vi "Control_motor.vi"() -> ()   [LabVIEW 2025]
uses:
  <vilib>/Instr/_visa.llb/VISA Configure Serial Port (Instr).vi
  <vilib>/addons/control/pid/pid.llb/PID (DBL).vi
  <vilib>/addons/control/pid/NI_PID_pid.lvlib
panel:
  out "Grados":dbl
  out "U":dbl format="%.2f"
  in  "Mandar Arduino":bool
  in  "Setpoint \nPosicion en grados":dbl
  in  "Kp":dbl=1.01
  in  "Ki":dbl=0.4
  in  "Kd":dbl=0.2
  in  "VISA resource name":refnum<visa-resource-name>
  out "Pulsos por vuelta":dbl
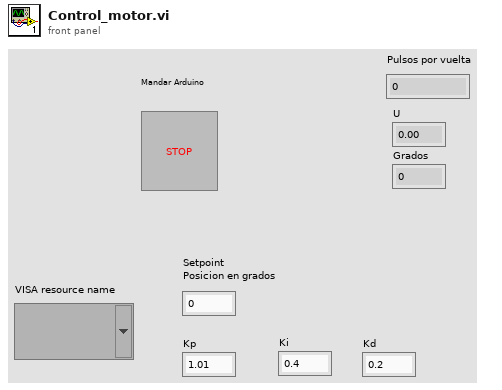
[diagram p1: front panel]
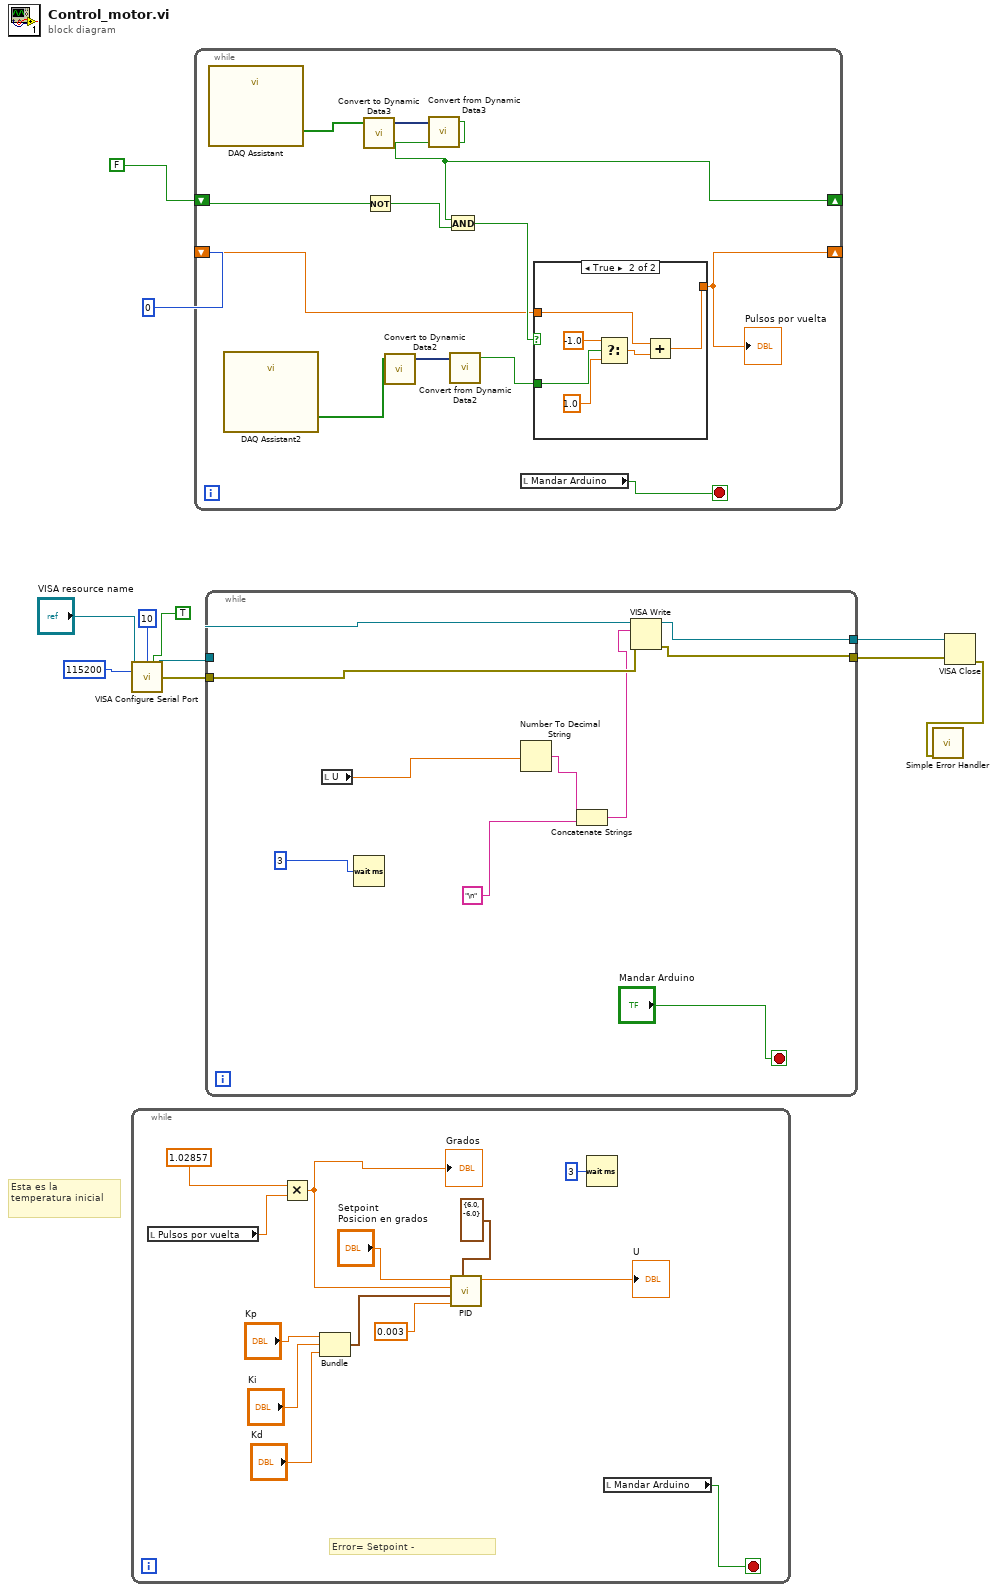
[diagram p0: block diagram]
diagram:
  # "Esta es la \ntemperatura inicial"
  n1 = call-poly "VISA Configure Serial Port"("VISA resource name"="VISA resource name", "termination char\n(0xA = '\\n' = LF)"=u8 10 ("termination char\n(0xA = '\\n' = LF)"), "Enable Termination\nChar (T)"=TRUE ("Enable Termination\nChar (T)"), "baud rate (9600)"=u32 115200) -> ("VISA resource name out"=w7:refnum<visa-resource-name>, "error out"=w6:errorcluster)  [unwired: 10 in]
  n2 = while {
    stop <- w12 stop-if-true
    # "Error= Setpoint -"
    n3 = local read "Pulsos por vuelta"() -> (w15:dbl)
    n4 = Multiply(x=1.02857, y=w15) -> (x*y=w13:dbl)
    "Grados" <- w13
    n5 = Bundle("Kp"="Kp", "Ki"="Ki", "Kd"="Kd") -> (w20:cluster{"Kp":dbl, "Ki":dbl, "Kd":dbl})  [unwired: 1 in]
    n6 = call-poly <vilib>:"PID.vi"("output range"=cluster{"output high":dbl, "output low":dbl} {"output high"=6.0, "output low"=-6.0}, "dt (s)"=0.003, "PID gains"=w20, "process variable"=w13, "setpoint"="Setpoint \nPosicion en grados") -> ("output"=→"U":dbl)  [unwired: 5 in, 1 out]
    n7 = Wait (ms)(milliseconds to wait=u32 3) -> ()  [unwired: 1 out]
    n8 = local read "Mandar Arduino"() -> (w12:bool)
  }
  n9 = while {
    shift-right: [w28] -> _
    shift-left: FALSE -> [w34]
    shift-right: [w32] -> _
    shift-left: 0 -> [w35]
    stop <- w25 stop-if-true
    n10 = call "DAQ Assistant"() -> ("data"=w27:bool[])  [unwired: 17 in, 2 out]
    n11 = call "DAQ Assistant2"() -> ("data"=w26:bool[])  [unwired: 17 in, 2 out]
    n12 = call "Convert to Dynamic Data3"("Array"=w27) -> ("Dynamic Data Type"=w29:dynamicdata)  [unwired: 3 in]
    n13 = Not(x=w34) -> (.not. x?=w33:bool)
    n14 = call "Convert to Dynamic Data2"("Array"=w26) -> ("Dynamic Data Type"=w31:dynamicdata)  [unwired: 3 in]
    n15 = call "Convert from Dynamic Data3"("Dynamic Data Type"=w29) -> ("Scalar"=w28:bool)  [unwired: 3 in]
    n16 = And(x=w28, y=w33) -> (x .and. y?=w36:bool)
    n17 = call "Convert from Dynamic Data2"("Dynamic Data Type"=w31) -> ("Scalar"=w30:bool)  [unwired: 3 in]
    n18 = local read "Mandar Arduino"() -> (w25:bool)
    n19 = case shown="True" w36 {
      tunnel: w30 -> [_ w43]
      tunnel: w35 -> [w37 w39]
      tunnel: [w37 w38] -> w32
      frame False {
      }
      frame True {
        n20 = Select(t=-1.0, s=w43, f=1.0) -> (s? t:f=w42:dbl)
        n21 = Add(x=w39, y=w42) -> (x+y=w38:dbl)
      }
    }
    "Pulsos por vuelta" <- w32
  }
  n22 = while {
    tunnel: w7 -> [w52]
    tunnel: w6 -> [w53]
    tunnel: [w50] -> w5
    tunnel: [w51] -> w4
    stop <- "Mandar Arduino" stop-if-true
    n23 = local read "U"() -> (w44:dbl)
    n24 = Wait (ms)(milliseconds to wait=u32 3) -> ()  [unwired: 1 out]
    n25 = Number To Decimal String(number=w44) -> (decimal integer string=w48:string)  [unwired: 1 in]
    n26 = Concatenate Strings(w48, "\n") -> (w47:string)
    n27 = VISA Write(VISA resource name=w52, write buffer=w47, error in (no error)=w53) -> (VISA resource name out=w51:refnum<visa-resource-name>, error out=w50:errorcluster)  [unwired: 1 out]
  }
  n28 = VISA Close(VISA resource name=w4, error in (no error)=w5) -> (error out=w3:errorcluster)
  n29 = call <vilib>:"Simple Error Handler.vi"("error in (no error)"=w3) -> ()  [unwired: 4 in, 5 out]
